vi "JSON to DAQ Configuration.vi"(8 "error in":errorcluster, 11 "flattened JSON configuration":string) -> (0 "error out":errorcluster, 3 "DAQmx Configuration":T1={"Run Mode"=0, "Sample Rate (Hz)"=51200.0, "Block Size"=5120, "Channel Table"=[], "Trigger Type"=0, "Trigger Channel"="", "Level"=1.0, "Pretrigger"=20, "Hysteresis"=0.0, "Slope"=enum."Rising"} {"Run Mode" items=["Run Once", "Continuously"]; "Block Size" min=0; "Sample Rate (Hz)" min=0.0; "Trigger Type" items=["None", "Analog Reference"]; "Channel Table"."input terminal configuration" items=["default"=-1, "RSE"=10083, "NRSE"=10078, "Differential"=10106, "Pseudodifferential"=12529]; "Channel Table"."Channel Type" items=["Voltage (V)"=0, "Charge (C)"=9, "-"=99, "SPL (Pa)"=3, "Force (lbf)"=6, "Force (N)"=1, "Acceleration (g) - IEPE"=2, "Acceleration (g) - Charge"=12, "Acceleration (g) - 4 wire DC Voltage"=22, "Velocity (in/s)"=7, "Velocity (mm/s)"=8, "Prox Probe (mil)"=4, "Prox Probe (mm)"=5]})   [LabVIEW 2024, in "Dynamic Signal Acquisition (Interactive) UI.lvlib"]
uses:
  Dynamic Signal Acquisition (Interactive) UI.lvlib
  SFPDAQ Configuration.ctl
  SFPDAQmx Channel Info.ctl
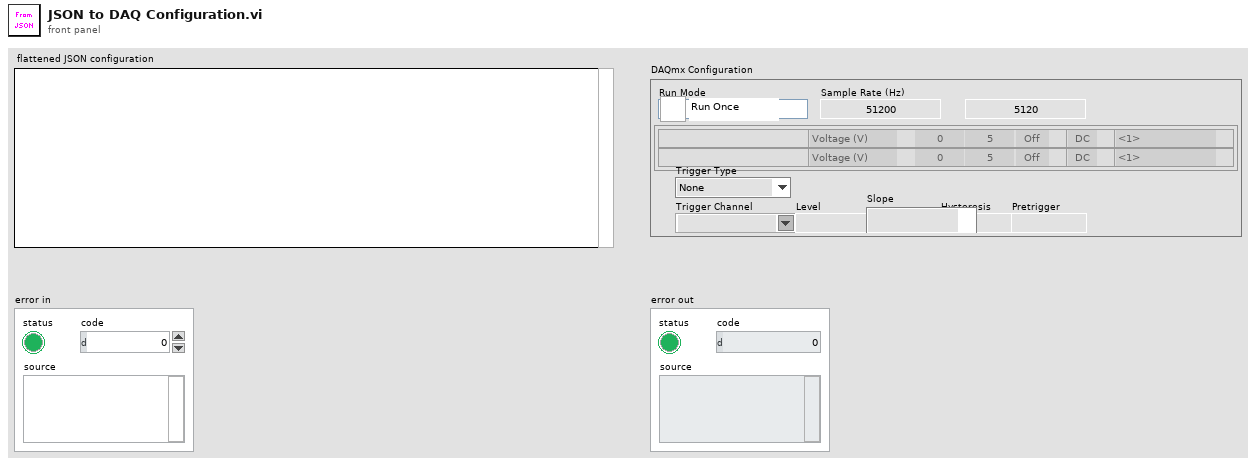
[diagram p1: front panel]
types:
  T1 = typedef "Dynamic Signal Acquisition (Interactive) UI.lvlib/SFPDAQ Configuration.ctl" = cluster{"Run Mode":u16, "Sample Rate (Hz)":dbl, "Block Size":i32, "Channel Table":T2[], "Trigger Type":u16, "Trigger Channel":string, "Level":dbl, "Pretrigger":i32, "Hysteresis":dbl, "Slope":enum16{"Falling", "Rising"}}
  T2 = typedef "Dynamic Signal Acquisition (Interactive) UI.lvlib/SFPDAQmx Channel Info.ctl" = cluster{"DAQmx Channel":tag, "Channel Type":u16, "Max":dbl, "Sensitivity":dbl, "Coupling":enum16{"AC", "DC"}, "input terminal configuration":i32, "excitation":enum16{"Off", "Min", "Max"}}
  T3 = cluster{"Sample Rate (Hz)":dbl, "Block Size":i32, "Channel Table":cluster{"DAQmx Channel":string, "Channel Type":u16, "Max":dbl, "Sensitivity":dbl, "Coupling":string, "input terminal configuration":i32, "excitation value":string}[], "Trigger Type":u16, "Trigger Channel":string, "Level":dbl, "Pretrigger":i32, "Hysteresis":dbl, "Slope":string, "Run Mode":u16}
  T4 = cluster{"DAQmx Channel":string, "Channel Type":u16, "Max":dbl, "Sensitivity":dbl, "Coupling":string, "input terminal configuration":i32, "excitation value":string}[]
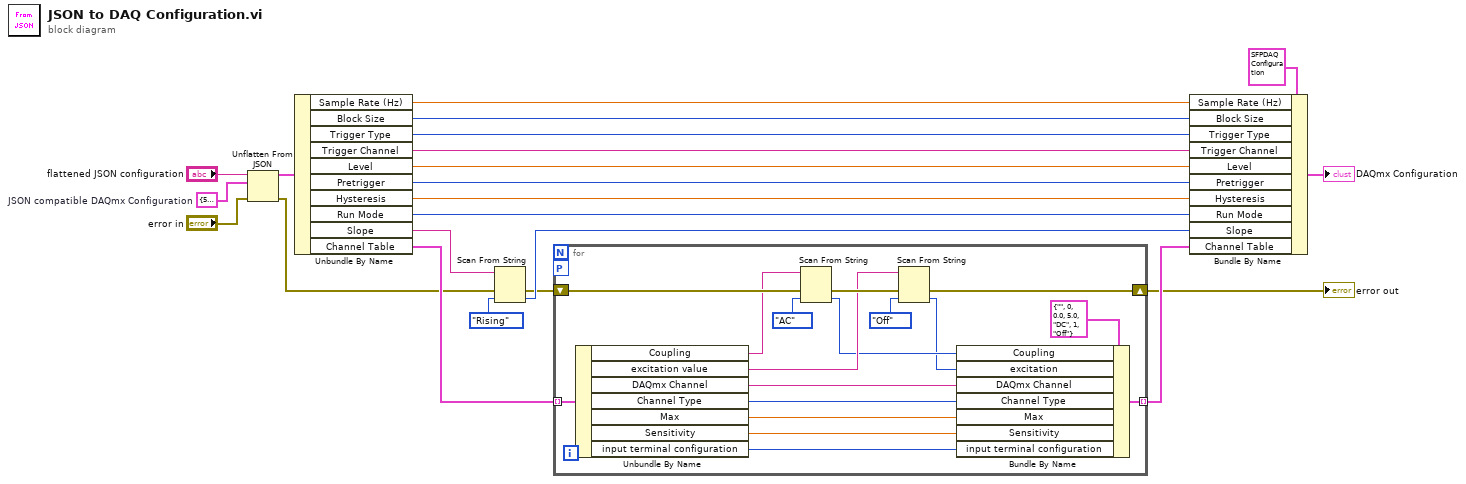
[diagram p0: block diagram]
diagram:
  w12 = T3 {"Sample Rate (Hz)"=51200.0, "Block Size"=5120, "Channel Table"=[], "Trigger Type"=0, "Trigger Channel"="", "Level"=0.0, "Pretrigger"=20, "Hysteresis"=0.0, "Slope"="", "Run Mode"=0}  # JSON compatible DAQmx Configuration
  n1 = Unflatten From JSON(JSON string="flattened JSON configuration", type and defaults=w12, error in (no error)="error in") -> (value=w11:T3, error out=w1:errorcluster)  [unwired: 4 in]
  n2 = Unbundle By Name(w11) -> ("Sample Rate (Hz)"=w21:dbl, "Block Size"=w20:i32, "Trigger Type"=w19:u16, "Trigger Channel"=w18:string, "Level"=w17:dbl, "Pretrigger"=w16:i32, "Hysteresis"=w15:dbl, "Run Mode"=w14:u16, "Slope"=w8:string, "Channel Table"=w22:T4)
  n3 = Scan From String(input string=w8, error in=w1, default 1=enum16{"Falling", "Rising"}."Rising" ("Slope")) -> (error out=w5:errorcluster, output 1=w6:enum16{"Falling", "Rising"})  [unwired: 2 in, 2 out]
  n4 = for {
    tunnel: w22 -> [w39] mode=indexing
    workers-P: _ -> [_]
    shift-right: [w23] -> w4
    shift-left: w5 -> [w31]
    tunnel: [w38] -> w9 mode=indexing
    n5 = Unbundle By Name(w39) -> ("Coupling"=w29:string, "excitation value"=w28:string, "DAQmx Channel"=w37:string, "Channel Type"=w36:u16, "Max"=w35:dbl, "Sensitivity"=w34:dbl, "input terminal configuration"=w33:i32)
    n6 = Scan From String(input string=w29, error in=w31, default 1=enum16{"AC", "DC"}."AC" ("Coupling")) -> (error out=w30:errorcluster, output 1=w26:enum16{"AC", "DC"})  [unwired: 2 in, 2 out]
    n7 = Scan From String(input string=w28, error in=w30, default 1=enum16{"Off", "Min", "Max"}."Off" ("excitation")) -> (error out=w23:errorcluster, output 1=w24:enum16{"Off", "Min", "Max"})  [unwired: 2 in, 2 out]
    n8 = Bundle By Name(cluster=T2 {"DAQmx Channel"="", "Channel Type"=0, "Max"=0.0, "Sensitivity"=5.0, "Coupling"=enum."DC", "input terminal configuration"=1, "excitation"=enum."Off"} ("Channel Information"), "Coupling"=w26, "excitation"=w24, "DAQmx Channel"=w37, "Channel Type"=w36, "Max"=w35, "Sensitivity"=w34, "input terminal configuration"=w33) -> (w38:T2)
  }
  "error out" <- w4
  n9 = Bundle By Name(cluster=T1 {"Run Mode"=0, "Sample Rate (Hz)"=51200.0, "Block Size"=5120, "Channel Table"=[], "Trigger Type"=0, "Trigger Channel"="", "Level"=1.0, "Pretrigger"=20, "Hysteresis"=0.0, "Slope"=enum."Rising"} ("DAQmx Configuration"), "Sample Rate (Hz)"=w21, "Block Size"=w20, "Trigger Type"=w19, "Trigger Channel"=w18, "Level"=w17, "Pretrigger"=w16, "Hysteresis"=w15, "Run Mode"=w14, "Slope"=w6, "Channel Table"=w9) -> (→"DAQmx Configuration":T1)
